vi "HEWH Check Power Set.vi"(6 "Station Data Output":T1={"Sequence #"=0.0, "Cycles"=0, "Mode Setting"="", "Flow Rate (GPM)"=0.0, "Temperature (F)"=0.0, "Reset Timer"=FALSE, "Use Temp Decline Method"=FALSE, "Terminate Condition"=enum."C1-Terminate Draw @ Gallon Mark", "Condition Value #1"=0.0, "UE"=FALSE, "LE"=FALSE, "Comp"=FALSE, "Fan"=FALSE, "Test End Time (Sec)"=0.0, "Purge Until Cutout"=FALSE, "Start Conditions"=enum."Heat Source Cutout", "Condition Value #2"=0.0, "Remove Power"=FALSE, "Time"=0.0, "Check Special Cond."=enum."SC2-Check Heat Source (On-C2/Off-C1)", "Condition#"=enum."C1", "Draw Flags"=enum."N/A", "Data Processing Delay (FHD 15sec, UEF 5 Sec)"=0.0, "Test Complete"=FALSE} {"Time" format="%<%H:%M:%S>t"}, 8 "Error In":errorcluster, 9 "Timer":dbl format="%<%H:%M:%S>t", 11 "HEWH Power":bool) -> (0 "Error Out":errorcluster, 2 "Set Power To This Value":bool, 3 "Trigger Power Set":bool)   [LabVIEW 2016]
uses:
  Type Definitions/PRAT Test.ctl
  Utility/Save File/File Setup (Public)/Type Definition/Save File HEWH Heating Control Mode.ctl
  Draw Water Specific/Type Definitions/Terminate Draw Conditions.ctl
  Type Definitions/HEWH Start Conditions.ctl
  Draw Water Specific/Type Definitions/Check Special Condtions.ctl
  Draw Water Specific/Type Definitions/HEWH Special Condition Check.ctl
  Type Definitions/HEWH Draw Flag ENUM.ctl
  Utility/Save File/File Setup.lvlib
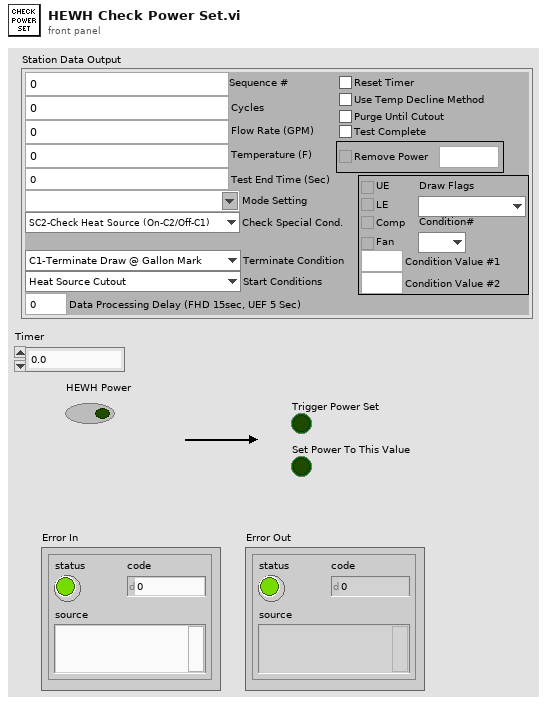
[diagram p1: front panel]
types:
  T1 = typedef "PRAT Test.ctl" = cluster{"Sequence #":dbl, "Cycles":i32, "Mode Setting":T2, "Flow Rate (GPM)":dbl, "Temperature (F)":dbl, "Reset Timer":bool, "Use Temp Decline Method":bool, "Terminate Condition":T3, "Condition Value #1":dbl, "UE":bool, "LE":bool, "Comp":bool, "Fan":bool, "Test End Time (Sec)":dbl, "Purge Until Cutout":bool, "Start Conditions":T4, "Condition Value #2":dbl, "Remove Power":bool, "Time":dbl, "Check Special Cond.":T5, "Condition#":T6, "Draw Flags":T7, "Data Processing Delay (FHD 15sec, UEF 5 Sec)":dbl, "Test Complete":bool}
  T2 = typedef "File Setup.lvlib/Save File HEWH Heating Control Mode.ctl" = string
  T3 = typedef "Terminate Draw Conditions.ctl" = enum16{"C1-Terminate Draw @ Gallon Mark", "C2-Special Last Draw (HU Test)", "C3-RTD Out <=", "C4-Mean Tank Temp <=", "C5-Decrease RTD Out (Deg F)", "C6-Time (Seconds)", "C7-Until Any Heat Source", "C8-Specific Heat Source", "C9-Do Nothing"}
  T4 = typedef "HEWH Start Conditions.ctl" = enum16{"Heat Source Cutout", "At Time (Seconds)", "Every X (Seconds)", "T2 >= X° Below Setpoint", "Seconds From Complete", "Wait for LE & Comp Cutout", "Wait for Comp Cutout", "Wait for LE Cutout", "Wait for UE Cutout"}
  T5 = typedef "Check Special Condtions.ctl" = enum16{"SC1-Do Nothing", "SC2-Check Heat Source (On-C2/Off-C1)", "SC3-Check Skip Condition", "SC4-Check Heat Source ON/Fail"}
  T6 = typedef "HEWH Special Condition Check.ctl" = enum16{"N/A", "C1", "C2", "Reset/Fail", "Skip Draw Sequence"}
  T7 = typedef "HEWH Draw Flag ENUM.ctl" = enum16{"N/A", "None(0)", "Sml(1)", "Med(2)", "SmlMed(3)", "Lrg(4)", "SmlLrg(5)", "MedLrg(6)", "SmlMedLrg(7)"}
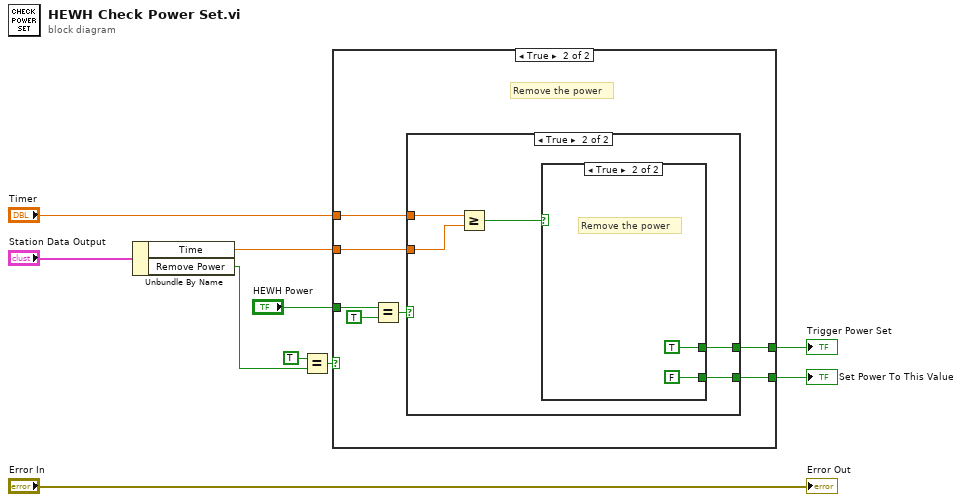
[diagram p0: block diagram]
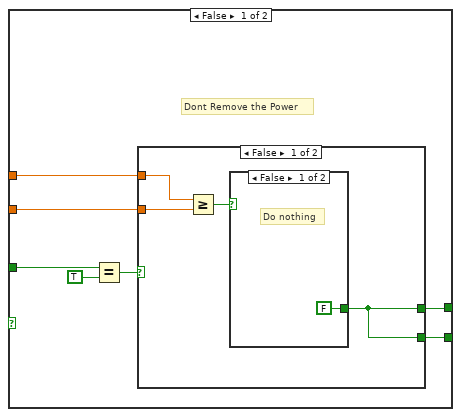
[diagram p2: hidden frame]
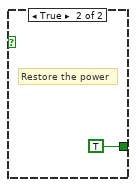
[diagram p3: hidden frame]
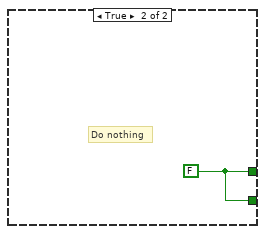
[diagram p4: hidden frame]
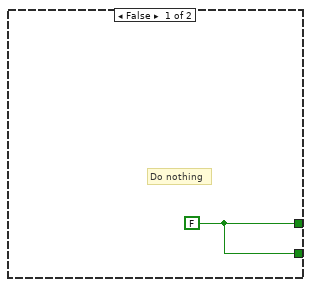
[diagram p5: hidden frame]
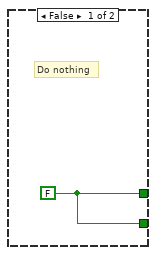
[diagram p6: hidden frame]
diagram:
  n1 = Unbundle By Name("Station Data Output") -> ("Time"=w2:dbl, "Remove Power"=w1:bool)
  n2 = Equal?(x=TRUE, y=w1) -> (x = y?=w9:bool)
  n3 = case shown="True" w9 {
    tunnel: "HEWH Power" -> [w16 w30]
    tunnel: [w14 w28] -> w7
    tunnel: [w13 w27] -> w6
    tunnel: "Timer" -> [w12 w26]
    tunnel: w2 -> [w11 w25]
    frame False {
      # "Dont Remove the Power"
      n4 = Equal?(x=w16, y=TRUE) -> (x = y?=w15:bool)
      n5 = case shown="False" w15 {
        tunnel: [w21 w24] -> w14
        tunnel: [w21 w24] -> w13
        tunnel: w12 -> [w20 _]
        tunnel: w11 -> [w19 _]
        frame False {
          n6 = Greater Or Equal?(x=w20, y=w19) -> (x >= y?=w18:bool)
          n7 = case shown="False" w18 {
            tunnel: [FALSE ("y") TRUE ("y")] -> w21
            frame False {
              # "Do nothing"
            }
            frame True {
              # "Restore the power"
            }
          }
        }
        frame True {
          w24 = FALSE ("y")
          # "Do nothing"
        }
      }
    }
    frame True {
      # "Remove the power"
      n8 = Equal?(x=w30, y=TRUE) -> (x = y?=w29:bool)
      n9 = case shown="True" w29 {
        tunnel: [w32 w34] -> w28
        tunnel: [w32 w33] -> w27
        tunnel: w26 -> [_ w37]
        tunnel: w25 -> [_ w36]
        frame False {
          w32 = FALSE ("Trigger Power Set")
          # "Do nothing"
        }
        frame True {
          n10 = Greater Or Equal?(x=w37, y=w36) -> (x >= y?=w35:bool)
          n11 = case shown="True" w35 {
            tunnel: [w38 TRUE ("Trigger Power Set")] -> w34
            tunnel: [w38 FALSE ("Trigger Power Set")] -> w33
            frame False {
              w38 = FALSE ("Trigger Power Set")
              # "Do nothing"
            }
            frame True {
              # "Remove the power"
            }
          }
        }
      }
    }
  }
  "Trigger Power Set" <- w7
  "Set Power To This Value" <- w6
  "Error Out" <- "Error In"
